vi "Set Controls and Indicators.vi"(6 "VI Index":i32, 10 "Controls":string[][](array[string]), 11 "VI Data":T1[](array[typedef])) -> (3 "VI Data out":T1[](array[typedef]))   [LabVIEW 2023, in "VI Properties Editor.lvlib"]
doc: "Sets all new control properties of the VI identified by <B>VI Index</B>."
uses:
  VI Properties Editor.lvlib
  CTLs/VI Data.ctl
  CTLs/VI Properties.ctl
  <vilib>/picture/picture.llb/imagedata.ctl
  CTLs/Control Properties.ctl
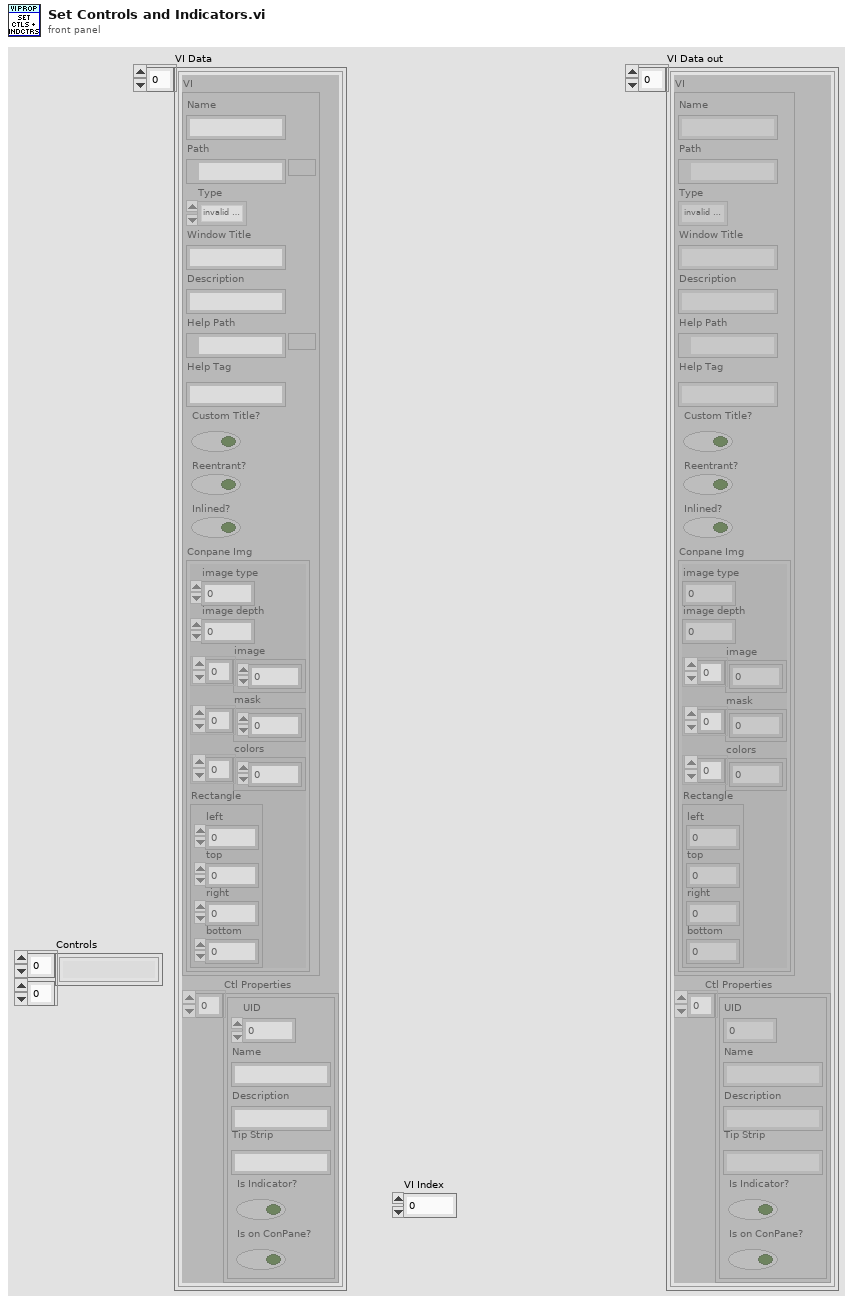
[diagram p1: front panel]
types:
  T1 = typedef "VI Properties Editor.lvlib/VI Data.ctl" = cluster{"VI":T2, "Ctl Properties":T4[]}
  T2 = typedef "VI Properties Editor.lvlib/VI Properties.ctl" = cluster{"Name":string, "Path":path, "Type":enum32{"invalid VI type", "Standard VI", "Control VI", "Global VI", "Polymorphic VI", "Configuration VI", "SubSystem", "Facade VI", "Method VI", "Statechart Diagram VI"}, "Window Title":string, "Description":string, "Help Path":path, "Help Tag":string, "Custom Title?":bool, "Reentrant?":bool, "Inlined?":bool, "Conpane Img":T3}
  T3 = typedef "imagedata.ctl" = cluster{"image type":i32, "image depth":i32, "image":u8[], "mask":u8[], "colors":u32[], "Rectangle":cluster{"left":i16, "top":i16, "right":i16, "bottom":i16}}
  T4 = typedef "VI Properties Editor.lvlib/Control Properties.ctl" = cluster{"UID":i32, "Name":string, "Description":string, "Tip Strip":string, "Is Indicator?":bool, "Is on ConPane?":bool}
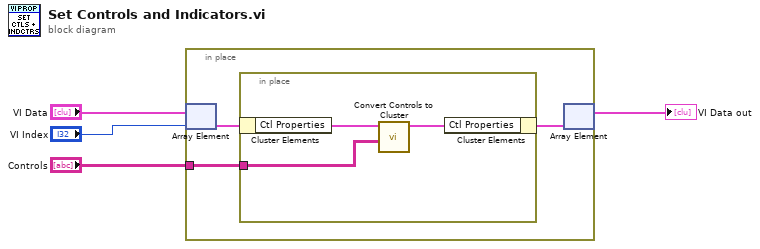
[diagram p0: block diagram]
diagram:
  n1 = in-place {
    in-place-border: "Controls" -> [w6]
    n2 = in-place-array #1("VI Data", "VI Index") -> (w7:T1)
    n3 = in-place {
      in-place-border: w6 -> [w8]
      n4 = in-place-cluster #2(w7) -> ("Ctl Properties"=w10:T4[])
      n5 = call "Convert Controls to Cluster.vi"("Control Array"=w8, "Ctl Properties"=w10) -> ("Ctl Properties out"=w9:T4[])  [unwired: 9 in]
      n6 = in-place-cluster #2("Ctl Properties"=w9) -> (w5:T1)
    }
    n7 = in-place-array #1(w5) -> (→"VI Data out":T1[])  [unwired: 1 out]
  }
